vi "CTRL_Send Cmd + DataString.vi"(0 "Port":refnum<visa-resource-name>, 5 "RS-485 addr.":u8, 7 "Cmd":T1="D", 9 "DataString":string, 11 "Error In":errorcluster) -> (4 "Port out":refnum<visa-resource-name>, 15 "Error Out":errorcluster)   [LabVIEW 2020]
uses:
  ctls/CTRL_Cmd.ctl
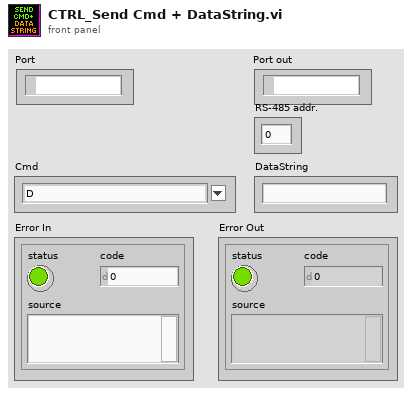
[diagram p1: front panel]
types:
  T1 = typedef "CTRL_Cmd.ctl" = string
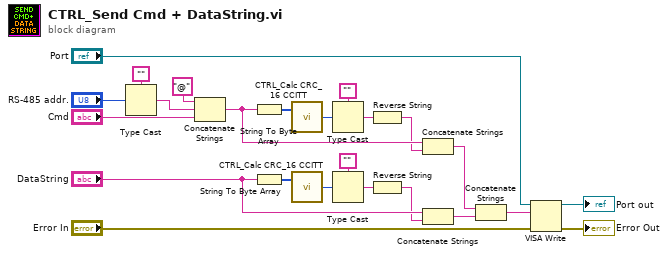
[diagram p0: block diagram]
diagram:
  n1 = Type Cast(type="", x="RS-485 addr.") -> (*(type *) &x=w16:string)
  n2 = Concatenate Strings("@", w16, "Cmd") -> (w11:string)
  n3 = String To Byte Array(string=w11) -> (unsigned byte array=w12:u8[])
  n4 = String To Byte Array(string="DataString") -> (unsigned byte array=w10:u8[])
  n5 = call "CTRL_Calc CRC_16 CCITT.vi"("Data bytes"=w12) -> ("CRC_16-CCITT"=w13:u16)  [unwired: 1 in]
  n6 = call "CTRL_Calc CRC_16 CCITT.vi"("Data bytes"=w10) -> ("CRC_16-CCITT"=w9:u16)  [unwired: 1 in]
  n7 = Type Cast(type="", x=w13) -> (*(type *) &x=w15:string)
  n8 = Type Cast(type="", x=w9) -> (*(type *) &x=w7:string)
  n9 = Reverse String(1:w15) -> (0:w1:string)
  n10 = Reverse String(1:w7) -> (0:w2:string)
  n11 = Concatenate Strings(w11, w1) -> (w5:string)
  n12 = Concatenate Strings("DataString", w2) -> (w4:string)
  n13 = Concatenate Strings(w5, w4) -> (w3:string)
  n14 = VISA Write(VISA resource name="Port", write buffer=w3, error in (no error)="Error In") -> (VISA resource name out=→"Port out":refnum<visa-resource-name>, error out=→"Error Out":errorcluster)  [unwired: 1 out]
